vi "test-trapezoid.vi"() -> ()   [LabVIEW 2016]
panel:
  out "Waveform Chart":dbl(graph)
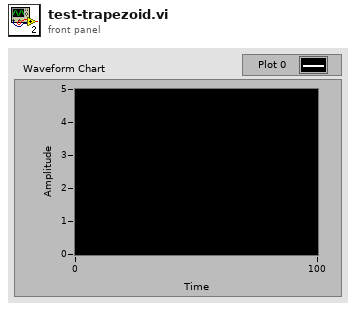
[diagram p1: front panel]
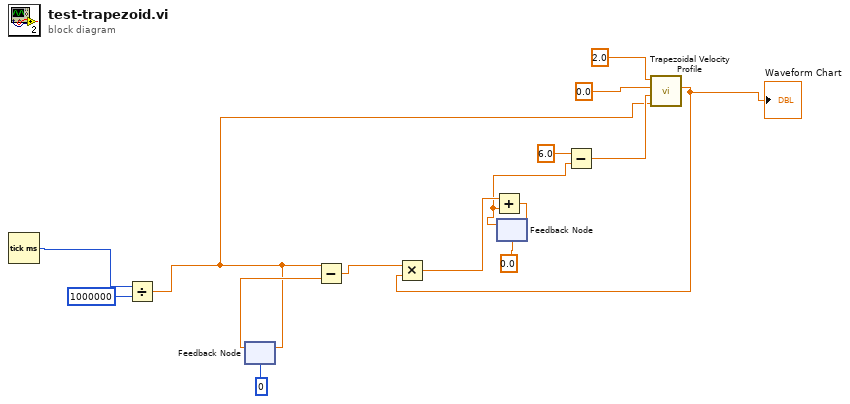
[diagram p0: block diagram]
diagram:
  n1 = Tick Count (ms)() -> (millisecond timer value=w1:u32)
  n2 = Divide(x=w1, y=u32 1000000) -> (x/y=w2:dbl)
  n3 = feedback-in #1(w2) -> ()
  n4 = feedback #1(u32 0 ("millisecond timer value")) -> (w10:dbl)
  n5 = Subtract(x=w2, y=w10) -> (x-y=w9:dbl)
  n6 = feedback #2(0.0) -> (w5:dbl)
  n7 = Subtract(x=6.0, y=w5) -> (x-y=w14:dbl)
  n8 = call "Trapezoidal Velocity Profile.vi"("t"=w2, "axis displacement (distance)"=w14, "initial velocity"=0.0, "set velocity"=2.0) -> ("velocity profile at t"=w4:dbl)  [unwired: 7 in]
  "Waveform Chart" <- w4
  n9 = Multiply(x=w9, y=w4) -> (x*y=w8:dbl)
  n10 = Add(x=w8, y=w5) -> (x+y=w7:dbl)
  n11 = feedback-in #2(w7) -> ()
